vi "RTM Writer Section Add Writer.vi"(8 "error in (no error)":errorcluster, 11 "Node Ptr":u64 format="%.0x") -> (0 "error out":errorcluster)   [LabVIEW 2015, in "DDS Custom Device System Explorer.lvlib"]
uses:
  DDS Custom Device System Explorer.lvlib
  Shared/Constants.vi
  Shared/DDS Custom Device Shared.lvlib
  <vilib>/NI VeriStand/Custom Device Tools/Custom Device Utility Library/Custom Device Utility Library.lvlib
  <vilib>/ni/NI VeriStand Advanced SysDef API/SysDef API/Advanced System Definition.lvlib
panel:
  in  "Tag":string
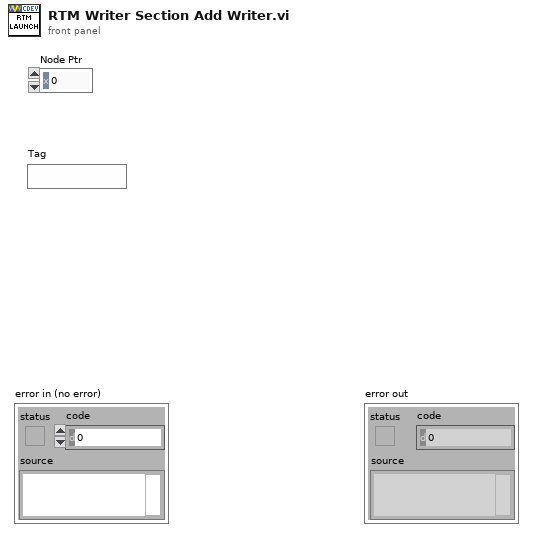
[diagram p1: front panel]
types:
  T1 = typedef "Custom Device API.lvlib/Custom Device Item Ref.ctl" = u64
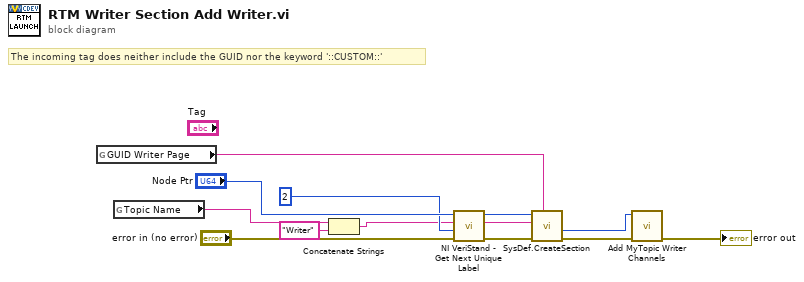
[diagram p0: block diagram]
diagram:
  # "The incoming tag does neither include the GUID nor the keyword '::CUSTOM::'"
  n1 = global read "Constants.vi" "GUID Writer Page"() -> (w4:string)
  n2 = global read "Constants.vi" "Topic Name"() -> (w10:string)
  n3 = Concatenate Strings(w10, "Writer" ("string")) -> (w8:string)
  n4 = call <vilib>:"NI VeriStand - Get Next Unique Label.vi"("error in (no error)"="error in (no error)", "Start Value (1)"=2, "Label"=w8, "Parent Ref in"="Node Ptr") -> ("error out"=w7:errorcluster, "Label out"=w6:string, "Parent Ref dup"=w5:T1)  [unwired: 4 in, 1 out]
  n5 = call <vilib>:"SysDef.CreateSection.vi"("GUID"=w4, "error in (no error)"=w7, "Name"=w6, "nodeID"=w5) -> ("error out"=w3:errorcluster, "New NodeID"=w1:u64)  [unwired: 4 in, 2 out]
  n6 = call "Add MyTopic Writer Channels.vi"("error in (no error)"=w3, "nodeID"=w1) -> ("error out"=→"error out":errorcluster)  [unwired: 8 in, 1 out]
